vi "PCAN Get LISTEN ONLY.vi"(7 "Language":T2 items=["System dependent", "Not available", "Not available", "Not available", "Not available", "Not available", "Not available", "Deutsch", "Not available", "English", "Español", "Not available", "Français", "Not available", "Not available", "Not available", "Italiano"], 8 "error in (no error)":errorcluster, 10 "TPCANParameter":T3=enum."PCAN listen-only" format="%x", 11 "TPCANHandle":T1) -> (0 "error out":errorcluster, 1 "Listen only Status":u32(ring) items=["PCAN_PARAMETER_OFF", "PCAN_PARAMETER_ON"], 3 "TPCANHandle out":T1)   [LabVIEW 2016]
doc: "Get PCAN_LISTEN_ONLY \n\nAccess: RW\n\nDescription: This parameter allows the user to set a CAN hardware in Listen-Only mode. When this mode is set, the CAN controller doens't take part on active events (eg. transmit CAN messages) but stays in a passive mode (CAN monitor), in which it can analyse the traffic on the CAN bus used by a PCAN channel. See also the Philips Data Sheet \"SJA1000 Stand-alone CAN controller\". \n\nPossible values: This parameter can have one of these values: PCAN_PARAMETER_OFF, PCAN_PARAMETER_ON. Note that other values will considered invalid. \n\nDefault value: Disabled (PCAN_PARAMETER_OFF). \n\nPCAN-Device: All PCAN devices containing a SJA1000 CAN controller."
uses:
  <instrlib>/KDI Digital Instrumentation/API_for_PCAN_BASIC_FD/TPCANHandle.ctl
  <instrlib>/KDI Digital Instrumentation/API_for_PCAN_BASIC_FD/TPCANParameter.ctl
  <instrlib>/KDI Digital Instrumentation/API_for_PCAN_BASIC_FD/Error language selector.ctl
  Users/MyUser/Documents/PCANBasic.dll
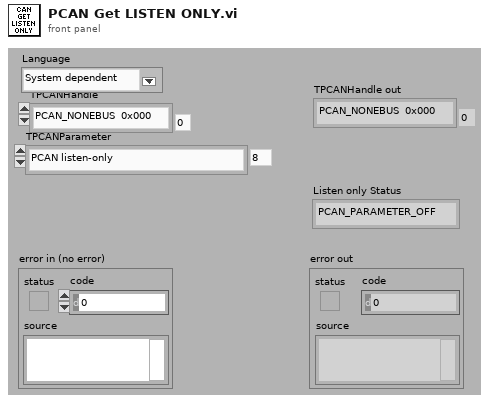
[diagram p1: front panel]
types:
  T1 = typedef "TPCANHandle.ctl" = enum16{"PCAN_NONEBUS  0x000", "PCAN_ISABUS1  0x21", "PCAN_ISABUS2  0x22", "PCAN_ISABUS3  0x23", "PCAN_ISABUS4  0x24", "PCAN_ISABUS5  0x25", "PCAN_ISABUS6  0x26", "PCAN_ISABUS7  0x27", "PCAN_ISABUS8  0x28", "PCAN_DNGBUS1  0x31", "PCAN_PCIBUS1  0x41", "PCAN_PCIBUS1  0x42", "PCAN_PCIBUS1  0x43", "PCAN_PCIBUS1  0x44", "PCAN_PCIBUS1  0x45", "PCAN_PCIBUS1  0x46", "PCAN_PCIBUS1  0x47", "PCAN_PCIBUS1  0x48", "PCAN_PCIBUS1  0x409", "PCAN_PCIBUS1  0x40A", "PCAN_PCIBUS1  0x40B", "PCAN_PCIBUS1  0x40C", "PCAN_PCIBUS1  0x40D", "PCAN_PCIBUS1  0x40E", "PCAN_PCIBUS1  0x40F", "PCAN_PCIBUS1  0x410", "PCAN_USBBUS1  0x51", "PCAN_USBBUS2  0x52", "PCAN_USBBUS3  0x53", "PCAN_USBBUS4  0x54", "PCAN_USBBUS5  0x55", "PCAN_USBBUS6  0x56", "PCAN_USBBUS7  0x57", "PCAN_USBBUS8  0x58", "PCAN_USBBUS9  0x509", "PCAN_USBBUS10  0x50A", "PCAN_USBBUS11  0x50B", "PCAN_USBBUS12  0x50C", "PCAN_USBBUS13  0x50D", "PCAN_USBBUS14  0x50E", "PCAN_USBBUS15  0x50F", "PCAN_USBBUS16  0x510", "PCAN_PCCBUS1  0x61", "PCAN_PCCBUS2  0x62", "PCAN_LANBUS1  0x801", "PCAN_LANBUS2  0x802", "PCAN_LANBUS3  0x803", "PCAN_LANBUS4  0x804", "PCAN_LANBUS5  0x805", "PCAN_LANBUS6  0x806", "PCAN_LANBUS7  0x807", "PCAN_LANBUS8  0x808", "PCAN_LANBUS9  0x809", "PCAN_LANBUS10  0x80A", "PCAN_LANBUS11  0x80B", "PCAN_LANBUS12  0x80C", "PCAN_LANBUS13  0x80D", "PCAN_LANBUS14  0x80E", "PCAN_LANBUS15  0x80F", "PCAN_LANBUS16  0x810"}
  T2 = typedef "Error language selector.ctl" = u16
  T3 = typedef "TPCANParameter.ctl" = enum8{"Not Available", "PCAN device number", "PCAN 5-volt power", "PCAN receive event", "PCAN message filter", "PCAN API version", "PCAN channel version", "PCAN busoff autoreset", "PCAN listen-only", "PCAN log location", "PCAN log status", "PCAN log configure", "PCAN log text", "PCAN channel condition", "PCAN hardware name", "PCAN_RECEIVE_STATUS", "PCAN_CONTROLLER_NUMBER", "PCAN_TRACE_LOCATION ", "PCAN_TRACE_STATUS", "PCAN_TRACE_SIZE", "PCAN_TRACE_CONFIGURE", "PCAN_CHANNEL_IDENTIFYING", "PCAN_CHANNEL_FEATURES", "PCAN_SPEED_ADAPTING", "PCAN_BITRATE_INFO", "PCAN_BITRATE_INFO_FD", "PCAN_BUSSPEED_NOMINAL", "PCAN_BUSSPEED_DATA", "PCAN_IP_ADDRESS", "PCAN_LAN_SERVICE_STATUS", "PCAN_ALLOW_STATUS_FRAMES", "PCAN_ALLOW_RTR_FRAMES", "PCAN_ALLOW_ERROR_FRAMES", "PCAN_INTERFRAME_DELAY", "PCAN_ACCEPTANCE_FILTER_11BIT", "PCAN_ACCEPTANCE_FILTER_29BIT", "PCAN_IO_DIGITAL_CONFIGURATION", "PCAN_IO_DIGITAL_VALUE", "PCAN_IO_DIGITAL_SET", "PCAN_IO_DIGITAL_CLEAR", "PCAN_IO_ANALOG_VALUE"}
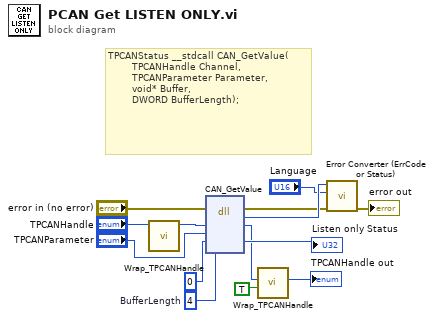
[diagram p0: block diagram]
diagram:
  w8 = u32 4  # BufferLength
  # "TPCANStatus __stdcall CAN_GetValue(\n        TPCANHandle Channel, \n        TPCANParameter Parameter,  \n        void* Buffer, \n        DWORD BufferLength);"
  n1 = call <instrlib>:"Wrap_TPCANHandle.vi"("TPCANHandle"="TPCANHandle") -> ("TPCANHandle out numeric"=w4:u16)  [unwired: 9 in, 1 out]
  n2 = dll-call lib="C:/Users/MyUser/Documents/PCANBasic.dll" fn="CAN_GetValue"(error in="error in (no error)", "TPCANHandle"=w4, "Parameter"="TPCANParameter", "Buffer"=u32 0, "BufferLength"=w8) -> (error out=w12:errorcluster, "return type"=w14:u32, "TPCANHandle"=w3:u16, "Buffer"=→"Listen only Status":u32)  [unwired: 4 in, 1 out]
  n3 = call <instrlib>:"Wrap_TPCANHandle.vi"("Wram num to enum"=TRUE, "TPCANHandle numeric"=w3) -> ("TPCANHandle out"=→"TPCANHandle out":T1)  [unwired: 8 in, 1 out]
  n4 = call <instrlib>:"Error Converter (ErrCode or Status).vi"("error in (no error)"=w12, "Language"="Language", "error code"=w14) -> ("error out"=→"error out":errorcluster)  [unwired: 8 in]
